vi "Config CDMA.vi"(0 "VISA Resource Name":refnum<visa-resource-name>, 1 "CDMA Select (1:9 CH FWD)":T2(ring)=enum."9 CH FWD", 2 "User CDMA State (CDMA_DATA)":string="CDMA_DATA", 3 "Chip Rate (1228800)":dbl=1228800.0 format="%.2f", 4 "Reconstruction Filter (1:2.5MHZ)":T1(ring)=enum."2.5 MHZ", 5 "error in (no error)":errorcluster {"code" format="%.0x"}, 6 "Waveform Length (1)":i32=1, 7 "Multicarrier (0: CAR3)":enum16{"CAR3", "CAR4", "CUSTOM"}(ring), 8 "Oversample Ratio (5)":i32=5, 10 "ARB Reference (F:INT)":bool, 12 "Reference Freq (10.0)":dbl=10.0 format="%.5f") -> (14 "VISA Resource Name Out":refnum<visa-resource-name>, 19 "error out":errorcluster {"code" format="%.0x"})   [LabVIEW 2014, in "Agilent ESG Series.lvlib"]
doc: "This VI is used to configure the CDMA option.\n\nNotes:\nThis VI is valid only on instruments with the UND and UN5 options or on instrument E4438C with option 401."
uses:
  Agilent ESG Series.lvlib
panel:
  # "EXT"
  # "INT"
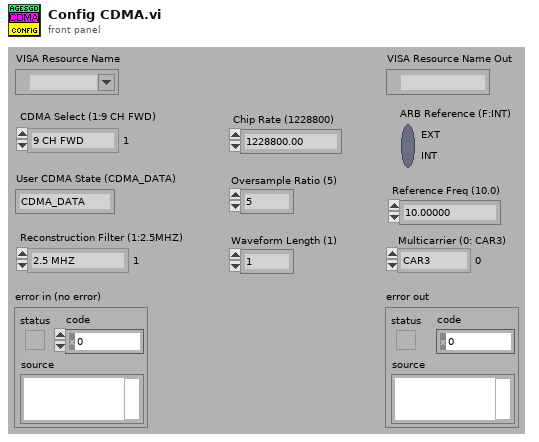
[diagram p1: front panel]
types:
  T1 = enum16{"250 KHZ", "2.5 MHZ", "8.0 MHZ", "THROUGH"}
  T2 = enum16{"PILOT", "9 CH FWD", "32 CH FWD", "64 CH FWD", "REVERSE", "CUSTOM", "MULTICARRIER"}
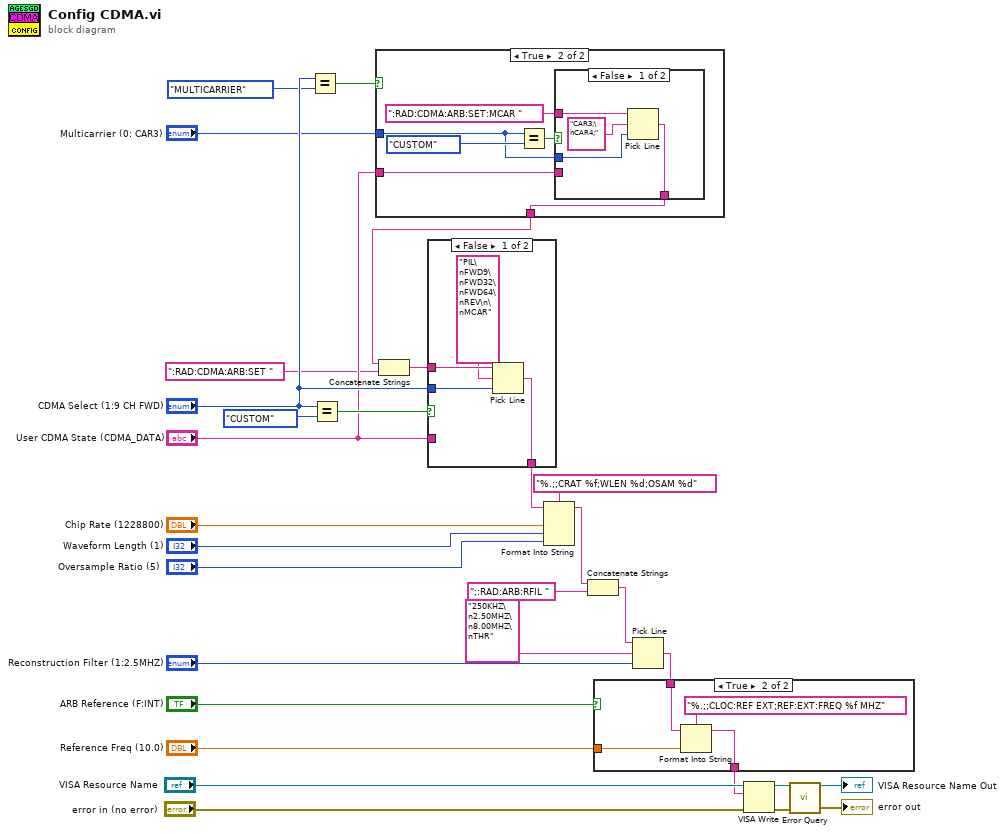
[diagram p0: block diagram]
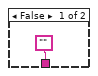
[diagram p2: hidden frame]
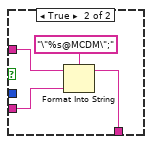
[diagram p3: hidden frame]
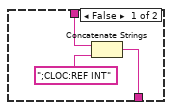
[diagram p4: hidden frame]
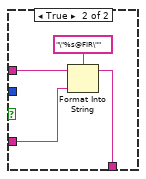
[diagram p5: hidden frame]
diagram:
  n1 = Equal?(x="CDMA Select (1:9 CH FWD)", y=T2."MULTICARRIER" ("CDMA Select (1:9 CH FWD)")) -> (x = y?=w10:bool)
  n2 = Equal?(x="CDMA Select (1:9 CH FWD)", y=T2."CUSTOM" ("CDMA Select (1:9 CH FWD)")) -> (x = y?=w28:bool)
  n3 = case shown="True" w10 {
    tunnel: ["" w34] -> w1
    tunnel: "Multicarrier (0: CAR3)" -> [_ w35]
    tunnel: "User CDMA State (CDMA_DATA)" -> [_ w33]
    frame False {
    }
    frame True {
      n4 = Equal?(x=w35, y=enum16{"CAR3", "CAR4", "CUSTOM"}."CUSTOM" ("Multicarrier (0: CAR3)")) -> (x = y?=w37:bool)
      n5 = case shown="False" w37 {
        tunnel: ":RAD:CDMA:ARB:SET:MCAR " ("string") -> [w41 w44]
        tunnel: w35 -> [w39 _]
        tunnel: [w38 w43] -> w34
        tunnel: w33 -> [_ w42]
        frame False {
          n6 = Pick Line(string ("")=w41, multi-line string="CAR3;\nCAR4;", line index=w39) -> (output string=w38:string)
        }
        frame True {
          n7 = Format Into String(format string="\"%s@MCDM\";", initial string=w44, w42) -> (resulting string=w43:string)  [unwired: 1 in, 1 out]
        }
      }
    }
  }
  n8 = Concatenate Strings(w1, ":RAD:CDMA:ARB:SET " ("string (\"\")")) -> (w3:string)
  n9 = case shown="False" w28 {
    tunnel: w3 -> [w49 w53]
    tunnel: "CDMA Select (1:9 CH FWD)" -> [w47 _]
    tunnel: [w46 w51] -> w4
    tunnel: "User CDMA State (CDMA_DATA)" -> [_ w50]
    frame False {
      n10 = Pick Line(string ("")=w49, multi-line string="PIL\nFWD9\nFWD32\nFWD64\nREV\n\nMCAR", line index=w47) -> (output string=w46:string)
    }
    frame True {
      n11 = Format Into String(format string="\"%s@FIR\"", initial string=w53, w50) -> (resulting string=w51:string)  [unwired: 1 in, 1 out]
    }
  }
  n12 = Format Into String(format string="%.;;CRAT %f;WLEN %d;OSAM %d", initial string=w4, "Chip Rate (1228800)", "Waveform Length (1)", "Oversample Ratio (5)") -> (resulting string=w25:string)  [unwired: 1 in, 1 out]
  n13 = Concatenate Strings(w25, ";:RAD:ARB:RFIL " ("string (\"\")")) -> (w21:string)
  n14 = Pick Line(string ("")=w21, multi-line string="250KHZ\n2.50MHZ\n8.00MHZ\nTHR", line index="Reconstruction Filter (1:2.5MHZ)") -> (output string=w22:string)
  n15 = case shown="True" "ARB Reference (F:INT)" {
    tunnel: w22 -> [w56 w60]
    tunnel: [w54 w57] -> w15
    tunnel: "Reference Freq (10.0)" -> [_ w58]
    frame False {
      n16 = Concatenate Strings(w56, ";CLOC:REF INT") -> (w54:string)
    }
    frame True {
      n17 = Format Into String(format string="%.;;CLOC:REF EXT;REF:EXT:FREQ %f MHZ", initial string=w60, w58) -> (resulting string=w57:string)  [unwired: 1 in, 1 out]
    }
  }
  n18 = VISA Write(VISA resource name="VISA Resource Name", write buffer=w15, error in (no error)="error in (no error)") -> (VISA resource name out=w14:refnum<visa-resource-name>, error out=w13:errorcluster)  [unwired: 1 out]
  n19 = call "Error Query.vi"("VISA Resource Name"=w14, "error in (no error)"=w13) -> ("VISA Resource Name Out"=→"VISA Resource Name Out":refnum<visa-resource-name>, "error out"=→"error out":errorcluster)  [unwired: 10 in, 2 out]
